vi "Get Next.vi"(0 "Parallel in":refnum<class "Parallel.lvclass">, 1 "Linked List Ref":refnum<data-value>, 5 "Active Unique ID":string, 9 "Active Element Index":i32, 11 "error in (no error)":errorcluster) -> (3 "Linked List Ref out":refnum<data-value>, 4 "Executioner out":refnum<class "Executioner.lvclass">, 6 "Active Unique ID out":string, 8 "Test Executive Ref out":refnum<data-value>, 10 "Active Element Index out":i32, 12 "Found":bool, 13 "Complete":bool, 14 "Stop":bool, 15 "error out":errorcluster)   [LabVIEW 2017, in "Custom Type Test Executive.lvlib" / "Parallel.lvclass"]
uses:
  <vilib>/gpm_packages/@cs/test-executive/Source/Custom Type Test Executive/Parallel/Parallel.lvclass
  C:/Program Files/National Instruments/LabVIEW 2017/vi.lib/gpm_packages/@cs/test-executive/Source/Test Executive/Parallel/Parallel.lvclass
  C:/Program Files/National Instruments/LabVIEW 2017/vi.lib/gpm_packages/@cs/test-executive/Source/Test Executive/Executioner/Executioner.lvclass
  <vilib>/gpm_packages/@cs/test-executive/Source/Test Executive/Executioner/Executioner.lvclass
  <vilib>/gpm_packages/@cs/linked-list/Source/Linked List/ILinkedList/ILinked List.lvclass
  <vilib>/gpm_packages/@cs/test-executive/Source/Test Executive/ITestExecutive/ITest Executive.lvclass
  <vilib>/gpm_packages/@cs/test-executive/Source/Custom Type Test Executive/Subroutine/Subroutine.lvclass
  <vilib>/gpm_packages/@cs/test-executive/Source/Custom Type Test Executive/Test Executive Data Type/Test Executive.lvclass/Test Executive.ctl
  <vilib>/gpm_packages/@cs/data-type-serializer/source/String/String.lvclass/String.ctl
  <vilib>/gpm_packages/@cs/test-executive/Source/Test Executive/Parallel/Parallel.lvclass/Parallel.ctl
  2094567f-b886-4e87-b085-7f7484cc6473.vi
  da8131fc-6b6d-43b6-aba5-ad3af7d3fec3.vi
  a64df0ad-f262-42a6-87d9-b37f8536d9fe.vi
  <vilib>/gpm_packages/@cs/test-executive/Source/Custom Type Test Executive/Test Executive Data Type/Test Executive.lvclass
  C:/Program Files/National Instruments/LabVIEW 2017/vi.lib/gpm_packages/@cs/data-type-serializer/source/Data Type/Data Type.lvclass
  <vilib>/gpm_packages/@cs/data-type-serializer/source/String/String.lvclass
  <vilib>/Utility/error.llb/Error Cluster From Error Code.vi
  <vilib>/gpm_packages/@cs/linked-list/Source/Linked List/Linked List Ref/Linked List Ref.lvclass
  <vilib>/gpm_packages/@cs/test-executive/Source/Test Executive/Parallel/Parallel.lvclass
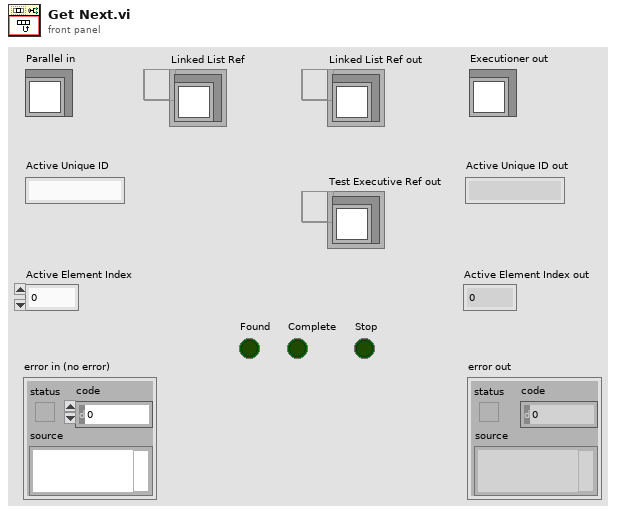
[diagram p1: front panel]
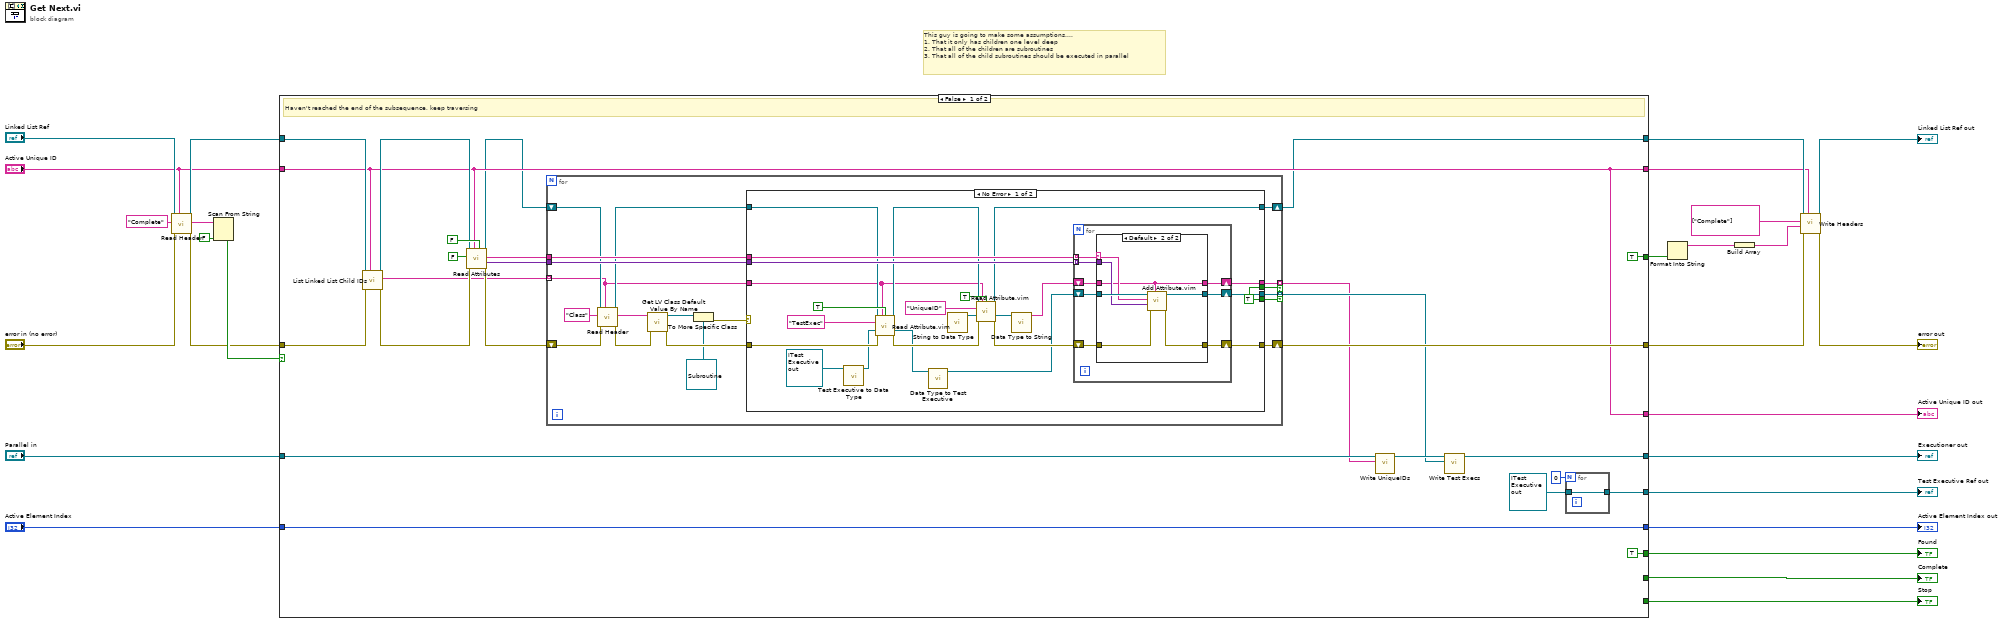
[diagram p0: block diagram]
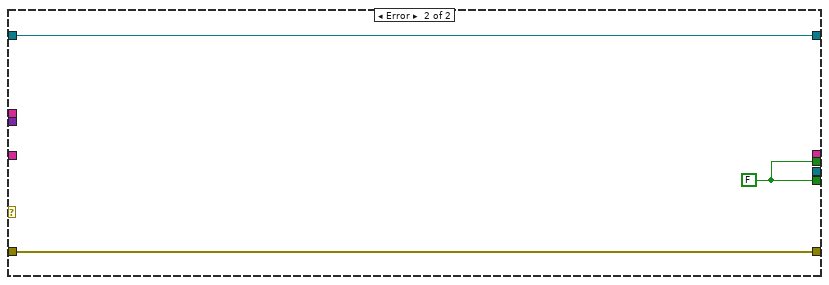
[diagram p3: hidden frame]
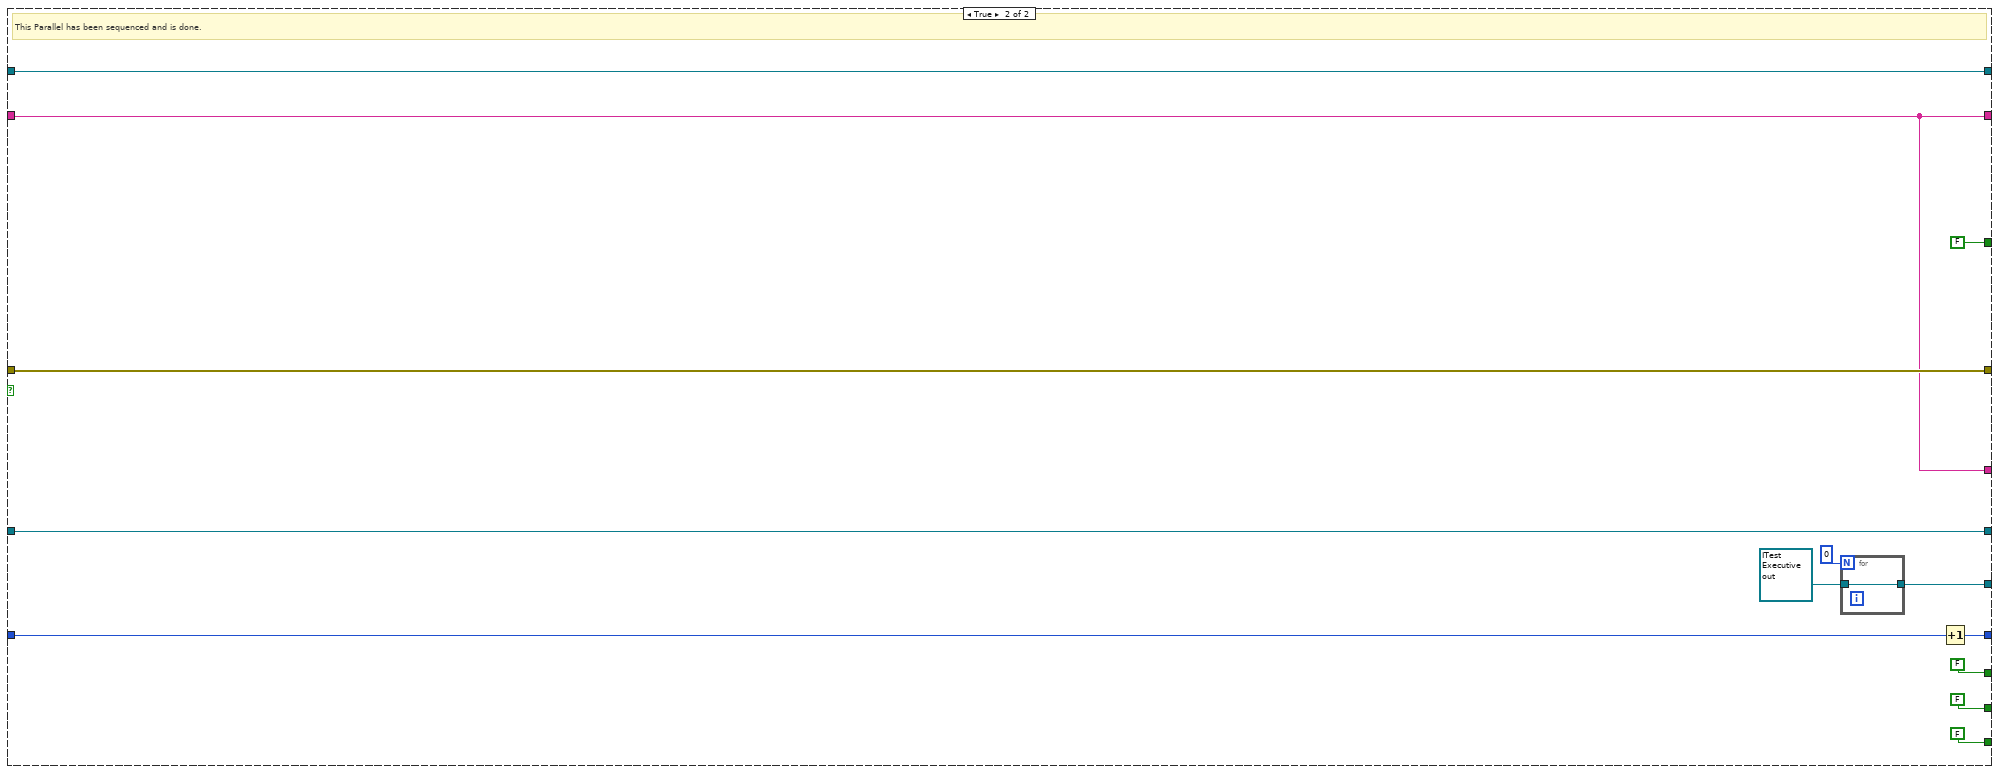
[diagram p4: hidden frame]
diagram:
  # "This guy is going to make some assumptions....\n1. That it only has children one level deep\n2. That all of the children are subroutines\n3. That all of the child subroutines should be executed in parallel"
  n1 = call <vilib>:"Read Header.vi"("Linked List ID"="Active Unique ID", "error in (no error)"="error in (no error)", "Header Name"="Complete" ("Attribute Name"), "Linked List Ref"="Linked List Ref") -> ("error out"=w15:errorcluster, "Header Value"=w19:string, "Linked List Ref out"=w16:refnum<data-value>)  [unwired: 4 in, 1 out]
  n2 = Scan From String(input string=w19, default 1=FALSE) -> (output 1=w17:bool)  [unwired: 3 in, 3 out]
  n3 = case shown="False" w17 {
    tunnel: [w33 w130] -> w27
    tunnel: w16 -> [w40 w130]
    tunnel: [w41 w129] -> w26
    tunnel: w15 -> [w38 w129]
    tunnel: "Active Element Index" -> [w52 w127]
    tunnel: [w36 w122] -> w25
    tunnel: "Active Unique ID" -> [w36 w122]
    tunnel: [w30 w128] -> w8
    tunnel: "Parallel in" -> [w32 w128]
    tunnel: [w52 w126] -> w6
    tunnel: [TRUE FALSE] -> w5
    tunnel: [_ FALSE] -> w2
    tunnel: [_ FALSE] -> w1
    tunnel: [w36 w122] -> w4
    tunnel: [TRUE FALSE] -> w24
    tunnel: [w47 w118] -> w7
    frame False {
      # "Haven't reached the end of the subsequence, keep traversing"
      n4 = call <vilib>:"List Linked List Child IDs.vi"("Linked List ID"=w36, "error in (no error)"=w38, "Linked List Ref"=w40) -> ("error out"=w37:errorcluster, "Child IDs"=w35:string[], "Linked List Ref out"=w39:refnum<data-value>)  [unwired: 6 in]
      n5 = call <vilib>:"Read Attributes.vi"("Flatten Pointer?"=FALSE, "Linked List ID"=w36, "error in (no error)"=w37, "Include Private?"=FALSE, "Linked List Ref"=w39) -> ("error out"=w45:errorcluster, "Attributes"=w42:variant[], "Attribute Names out"=w44:string[], "Linked List Ref out"=w34:refnum<data-value>)  [unwired: 1 in, 2 out]
      n6 = for {
        tunnel: w44 -> [w71]
        tunnel: w42 -> [w70]
        shift-right: [w69] -> w41
        shift-left: w45 -> [w64]
        tunnel: [w68] -> w28 mode=indexing if=w55
        tunnel: [w67] -> w29 mode=indexing if=w54
        tunnel: w35 -> [w58] mode=indexing
        shift-right: [w59] -> w33
        shift-left: w34 -> [w65]
        n7 = call <vilib>:"Read Header.vi"("Linked List ID"=w58, "error in (no error)"=w64, "Header Name"="Class", "Linked List Ref"=w65) -> ("error out"=w62:errorcluster, "Header Value"=w63:string, "Linked List Ref out"=w60:refnum<data-value>)  [unwired: 4 in, 1 out]
        n8 = call <vilib>:"Get LV Class Default Value By Name.vi"("error in (no error)"=w62, "class name"=w63) -> ("error out"=w57:errorcluster, "object"=w61:refnum<class>)  [unwired: 8 in]
        n9 = To More Specific Class(target class=refnum<class "Subroutine.lvclass"> refnum ("Custom Type Test Executive.lvlib:Subroutine.lvclass"), reference=w61) -> (error out=w56:errorcluster)  [unwired: 1 in, 1 out]
        n10 = case shown="No Error" w56 {
          tunnel: w71 -> [w95 _]
          tunnel: w70 -> [w94 _]
          tunnel: [w93 w115] -> w69
          tunnel: [w92 _] -> w68
          tunnel: [w91 _] -> w67
          tunnel: w60 -> [w85 w116]
          tunnel: [w83 w116] -> w59
          tunnel: w58 -> [w82 _]
          tunnel: w57 -> [w81 w115]
          tunnel: [w79 w114] -> w55
          tunnel: [w79 w114] -> w54
          frame No Error {
            w79 = TRUE
            n11 = call <vilib>:"Test Executive to Data Type.vi"("Test Executive Ref"=refnum<data-value> refnum ("Test Executive Ref out")) -> ("Boolean out"=w77:refnum<class "Test Executive.lvclass">)  [unwired: 9 in, 1 out]
            n12 = call "Read Attribute.vim"("Linked List Ref"=w85, "Linked List ID"=w82, "Include Private?"=TRUE, "Attribute Name"="TestExec", "Type"=w77, "error in (no error)"=w81) -> ("Linked List Ref out"=w84:refnum<data-value>, "Attribute"=w76:refnum<class "Test Executive.lvclass">, "error out"=w87:errorcluster)  [unwired: 4 in, 3 out]
            n13 = call <vilib>:"Data Type to Test Executive.vi"("Data Type"=w76) -> ("Test Executive Ref"=w75:refnum<data-value>)  [unwired: 9 in, 1 out]
            n14 = call <vilib>:"String to Data Type.vi"() -> ("Boolean out"=w74:refnum<class "String.lvclass">)  [unwired: 10 in, 1 out]
            n15 = call "Read Attribute.vim"("Linked List Ref"=w84, "Linked List ID"=w82, "Include Private?"=TRUE, "Attribute Name"="UniqueID", "Type"=w74, "error in (no error)"=w87) -> ("Linked List Ref out"=w83:refnum<data-value>, "Attribute"=w73:refnum<class "String.lvclass">, "error out"=w80:errorcluster)  [unwired: 4 in, 3 out]
            n16 = call <vilib>:"Data Type to String.vi"("Data Type"=w73) -> ("String out"=w72:string)  [unwired: 9 in, 1 out]
            n17 = for {
              shift-right: [w100] -> w93
              shift-left: w80 -> [w101]
              tunnel: w95 -> [w99] mode=indexing
              tunnel: w94 -> [w98] mode=indexing
              shift-right: [w97] -> w92
              shift-left: w72 -> [w102]
              shift-right: [w96] -> w91
              shift-left: w75 -> [w103]
              n18 = case shown="Default" w99 {
                selector: w99 -> [_ w110]
                tunnel: w103 -> [w104 w113]
                tunnel: w102 -> [w105 w108]
                tunnel: w101 -> [w106 w112]
                tunnel: [w106 w111] -> w100
                tunnel: w98 -> [_ w109]
                tunnel: [w105 w108] -> w97
                tunnel: [w104 w107] -> w96
                frame "Restore Point" {
                }
                frame Default {
                  n19 = call "Add Attribute.vim"("ID"=w108, "error in (no error)"=w112, "Attribute"=w109, "Attribute Name"=w110, "Test Executive Ref"=w113) -> ("error out"=w111:errorcluster, "Test Executive Ref out"=w107:refnum<data-value>)  [unwired: 3 in, 2 out]
                }
              }
            }
          }
          frame Error {
            w114 = FALSE
          }
        }
      }
      n20 = call <vilib>:"Write UniqueIDs.vi"("UniqueIDs"=w28, "Parallel in"=w32) -> ("Parallel out"=w31:refnum<class "Parallel.lvclass">)  [unwired: 9 in]
      n21 = call <vilib>:"Write Test Execs.vi"("Test Execs"=w29, "Parallel in"=w31) -> ("Parallel out"=w30:refnum<class "Parallel.lvclass">)  [unwired: 9 in]
      n22 = for {
        N: 0 -> [_]
        tunnel: refnum<data-value> refnum ("Test Executive Ref out") -> [w117]
        tunnel: [w117] -> w47
      }
    }
    frame True {
      # "This Parallel has been sequenced and is done."
      n23 = for {
        N: 0 -> [_]
        tunnel: refnum<data-value> refnum ("Test Executive Ref out") -> [w131]
        tunnel: [w131] -> w118
      }
      n24 = Increment(x=w127) -> (x+1=w126:i32)
    }
  }
  "Executioner out" <- w8
  "Active Unique ID out" <- w4
  "Active Element Index out" <- w6
  "Found" <- w5
  "Complete" <- w2
  "Stop" <- w1
  "Test Executive Ref out" <- w7
  n25 = Format Into String(w24) -> (resulting string=w22:string)  [unwired: 3 in, 1 out]
  n26 = Build Array(w22) -> (w21:string[])
  n27 = call <vilib>:"Write Headers.vi"("Linked List ID"=w25, "error in (no error)"=w26, "Header Values"=w21, "Header Names"=string[] ["Complete"], "Linked List Ref"=w27) -> ("error out"=→"error out":errorcluster, "Linked List Ref out"=→"Linked List Ref out":refnum<data-value>)  [unwired: 5 in]
